vi "Generate Server RPC Methods.vi"(7 "RPC Method Parameters":T1[](array[typedef]), 8 "error in (no error)":errorcluster, 10 "Library":refnum<vi>, 11 "Server class in":refnum<vi>) -> (0 "error out":errorcluster, 2 "Newly created methods count":i64, 3 "Server class out":refnum<vi>)   [LabVIEW 2019, in "gRPC Template Creation Utility.lvlib"]
uses:
  gRPC Template Creation Utility.lvlib
  TypeDefs/RPC Method Parameters.ctl
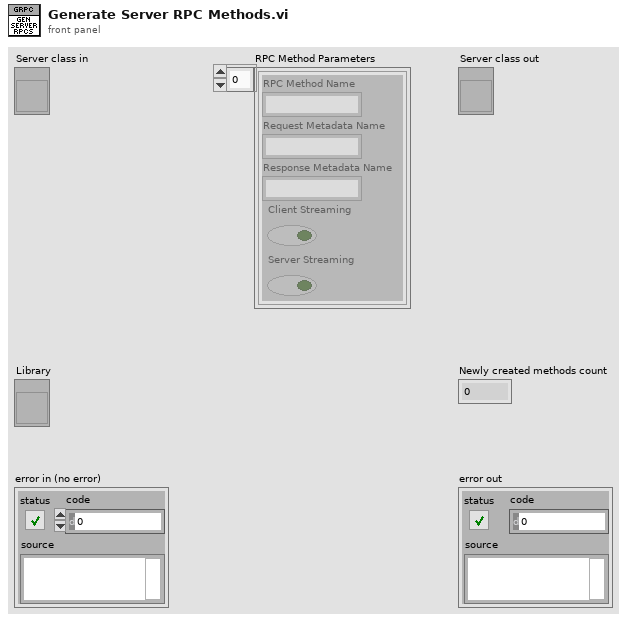
[diagram p1: front panel]
types:
  T1 = typedef "gRPC Template Creation Utility.lvlib/RPC Method Parameters.ctl" = cluster{"RPC Method Name":string, "Request Metadata Name":string, "Response Metadata Name":string, "Client Streaming":bool, "Server Streaming":bool}
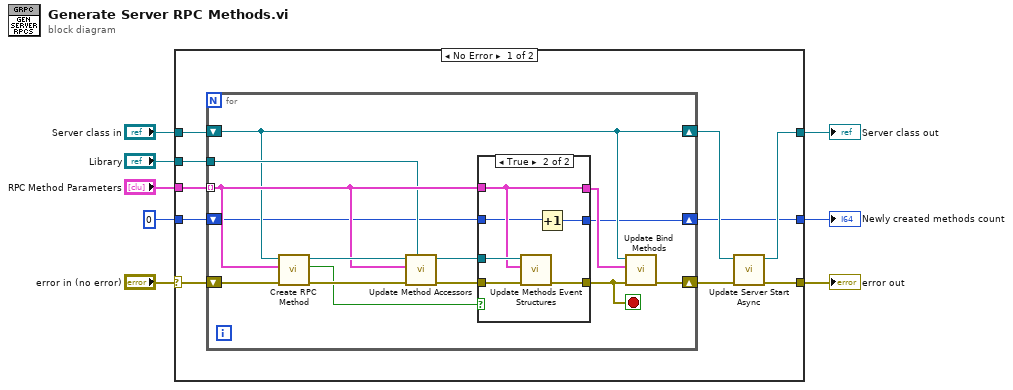
[diagram p0: block diagram]
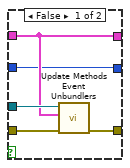
[diagram p2: hidden frame]
diagram:
  n1 = case shown="No Error" "error in (no error)" {
    selector: "error in (no error)" -> [w18 w46]
    tunnel: [w15 w46] -> w8
    tunnel: "Server class in" -> [w17 w45]
    tunnel: [w14 w45] -> w5
    tunnel: "RPC Method Parameters" -> [w16 _]
    tunnel: "Library" -> [w13 _]
    tunnel: i64 0 -> [w10 w44]
    tunnel: [w9 w44] -> w1
    frame No Error {
      n2 = for {
        tunnel: w16 -> [w27] mode=indexing
        shift-right: [w23] -> w12
        shift-left: w18 -> [w32]
        shift-right: [w21] -> w11
        shift-left: w17 -> [w21]
        tunnel: w13 -> [w25]
        shift-right: [w19] -> w9
        shift-left: w10 -> [w20]
        stop <- w24 stop-if-true
        n3 = call "Create RPC Method.vi"("error in (no error)"=w32, "rpc method parameters"=w27, "server class in"=w21) -> ("error out"=w29:errorcluster, "newly created ?"=w26:bool, "server class out"=w31:refnum<vi>)  [unwired: 6 in]
        n4 = call "Update Method Accessors.vi"("Library"=w25, "error in (no error)"=w29, "RPC Method Parameters"=w27, "Server class in"=w31) -> ("error out"=w28:errorcluster, "Server class out"=w30:refnum<vi>)  [unwired: 6 in]
        n5 = case shown="True" w26 {
          tunnel: w28 -> [w37 w43]
          tunnel: w30 -> [w35 w42]
          tunnel: w27 -> [w34 w40]
          tunnel: [w36 w41] -> w24
          tunnel: [w34 w40] -> w22
          tunnel: w20 -> [w33 w39]
          tunnel: [w33 w38] -> w19
          frame False {
            n6 = call "Update Methods Event Unbundlers.vi"("error in (no error)"=w37, "RPC Method Parameters"=w34, "LVClassLibrary in"=w35) -> ("error out"=w36:errorcluster)  [unwired: 7 in, 1 out]
          }
          frame True {
            n7 = call "Update Methods Event Structures.vi"("error in (no error)"=w43, "RPC Method Parameters"=w40, "LVClassLibrary in"=w42) -> ("error out"=w41:errorcluster)  [unwired: 7 in, 1 out]
            n8 = Increment(x=w39) -> (x+1=w38:i64)
          }
        }
        n9 = call "Update Bind Methods.vi"("error in (no error)"=w24, "RPC Method Parameters"=w22, "Server class in"=w21) -> ("error out"=w23:errorcluster)  [unwired: 7 in, 1 out]
      }
      n10 = call "Update Server Start Async.vi"("error in (no error)"=w12, "Server class in"=w11) -> ("error out"=w15:errorcluster, "Server class out"=w14:refnum<vi>)  [unwired: 8 in]
    }
    frame Error {
    }
  }
  "error out" <- w8
  "Server class out" <- w5
  "Newly created methods count" <- w1
